vi "From CSV File.vi"(8 "error in (no error)":errorcluster, 9 "Path":path, 10 "engine in":refnum<class "engine configuration.lvclass">, 11 "Modbus Module editor node in":refnum<class "Modbus Module editor node.lvclass">) -> (0 "error out":errorcluster, 1 "Update":bool, 2 "engine out":refnum<class "engine configuration.lvclass">, 3 "Modbus Module editor node out":refnum<class "Modbus Module editor node.lvclass">)   [LabVIEW 2015, in "Modbus Module editor node.lvclass"]
uses:
  Modbus Module editor node.lvclass
  <vilib>/NI/Module Execution Interface/Engine Configuration/engine configuration.lvclass
  module/configuration/Modbus Module configuration.lvclass
  <vilib>/NI/Configuration Framework/serializable configuration/NISE_CEF_serializable configuration.lvclass/NISE_CEF_serializable configuration.ctl
  <vilib>/Utility/LVClass/Get LV Class Name.vi
  <vilib>/NI/Configuration Framework/error generator/NISE_error generator.vi
  <vilib>/NI/Configuration Framework/serializable configuration/NISE_CEF_serializable configuration.lvclass
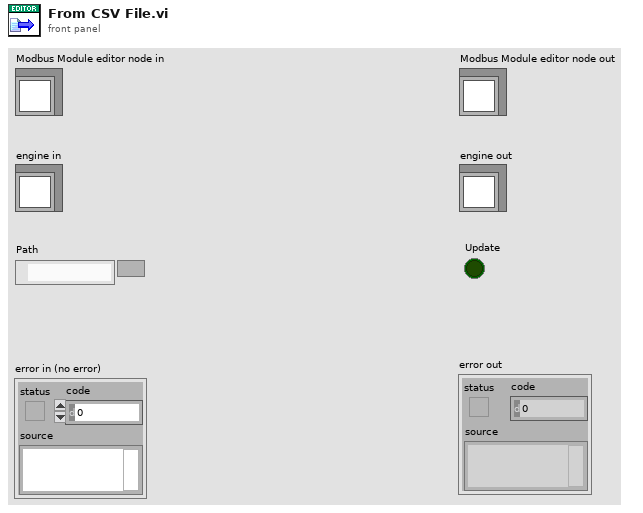
[diagram p1: front panel]
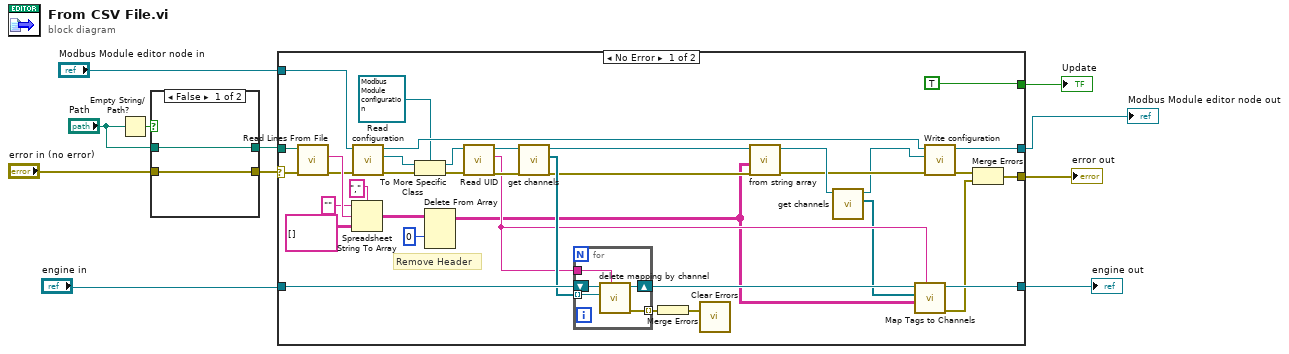
[diagram p0: block diagram]
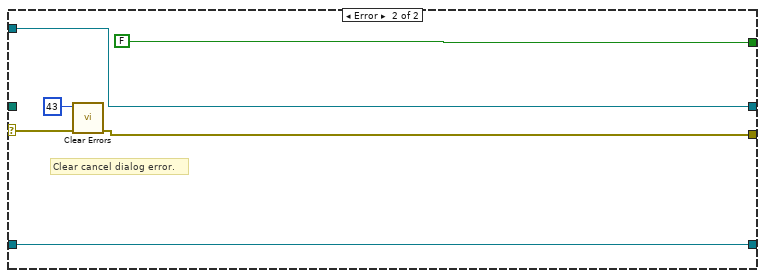
[diagram p2: hidden frame]
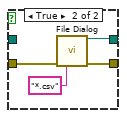
[diagram p3: hidden frame]
diagram:
  n1 = Empty String/Path?(string/path="Path") -> (empty?=w11:bool)
  n2 = case shown="False" w11 {
    tunnel: "error in (no error)" -> [w13 w16]
    tunnel: [w13 w15] -> w9
    tunnel: [w12 w14] -> w10
    tunnel: "Path" -> [w12 _]
    frame False {
    }
    frame True {
      n3 = call "File Dialog"("error in"=w16, "pattern (all files)"="*.csv") -> ("selected path"=w14:path, "error out"=w15:errorcluster)  [unwired: 10 in, 2 out]
    }
  }
  n4 = case shown="No Error" w9 {
    selector: w9 -> [w47 w62]
    tunnel: [w39 w61] -> w2
    tunnel: [w33 w64] -> w5
    tunnel: "Modbus Module editor node in" -> [w38 w64]
    tunnel: w10 -> [w52 _]
    tunnel: [TRUE ("Update") FALSE ("Update")] -> w3
    tunnel: "engine in" -> [w44 w59]
    tunnel: [w25 w59] -> w4
    frame No Error {
      # "Remove Header"
      n5 = call <vilib>:"Read Lines From File.vi"("file path (dialog if empty)"=w52, "error in (not an error)"=w47) -> ("line string"=w50:string, "error out"=w37:errorcluster)  [unwired: 5 in, 1 out]
      n6 = Spreadsheet String To Array(delimiter (Tab)=",", format string="", spreadsheet string=w50, array type (2D Dbl)=string[][] [] ("type (empty)")) -> (array=w20:string[][])
      n7 = call-dynamic "Read configuration.vi"("error in"=w37, "Modbus Slave editor node in"=w38) -> ("error out"=w35:errorcluster, "configuration"=w36:refnum<class "NISE_CEF_serializable configuration.lvclass">, "Modbus Slave editor node out"=w34:refnum<class "Modbus Module editor node.lvclass">)  [unwired: 7 in]
      n8 = To More Specific Class(target class=refnum<class "Modbus Module configuration.lvclass"> refnum ("Modbus Module configuration"), reference=w36, error in=w35) -> (specific class reference=w46:refnum<class "Modbus Module configuration.lvclass">, error out=w40:errorcluster)
      n9 = Delete From Array(array=w20, index (row)=0) -> (array with subset deleted=w19:string[][])  [unwired: 2 in, 1 out]
      n10 = call <vilib>:"Read UID.vi"("error in"=w40, "configuration in"=w46) -> ("error out"=w30:errorcluster, "instance id"=w22:string, "configuration out"=w45:refnum<class "Modbus Module configuration.lvclass">)  [unwired: 7 in]
      n11 = call-dynamic "get channels.vi"("Modbus Slave configuration in"=w45) -> ("channels"=w43:refnum<class "TBM channel.lvclass">[], "Modbus Slave configuration out"=w41:refnum<class "Modbus Module configuration.lvclass">)  [unwired: 9 in]
      n12 = for {
        tunnel: w22 -> [w57]
        tunnel: w43 -> [w56] mode=indexing
        tunnel: [w55] -> w42 mode=indexing
        shift-right: [w54] -> w24
        shift-left: w44 -> [w58]
        n13 = call <vilib>:"delete mapping by channel.vi"("owner ID"=w57, "channel"=w56, "engine configuration in"=w58) -> ("error out"=w55:errorcluster, "engine configuration out"=w54:refnum<class "engine configuration.lvclass">)  [unwired: 7 in]
      }
      n14 = Merge Errors(w42) -> (w31:errorcluster)
      n15 = call <vilib>:"Clear Errors.vi"("error in (no error)"=w31) -> ()  [unwired: 5 in, 2 out]
      n16 = call-dynamic "from string array.vi"("error in (no error)"=w30, "String Array"=w19, "module configuration in"=w41) -> ("error out"=w27:errorcluster, "module configuration out"=w28:refnum<class "Modbus Module configuration.lvclass">)  [unwired: 7 in]
      n17 = call-dynamic "get channels.vi"("Modbus Slave configuration in"=w28) -> ("channels"=w21:refnum<class "TBM channel.lvclass">[], "Modbus Slave configuration out"=w26:refnum<class "Modbus Module configuration.lvclass">)  [unwired: 9 in]
      n18 = call "Map Tags to Channels.vi"("instance id"=w22, "String Array"=w19, "channels"=w21, "engine configuration in"=w24) -> ("error out"=w23:errorcluster, "engine configuration out"=w25:refnum<class "engine configuration.lvclass">)  [unwired: 6 in]
      n19 = call-dynamic "Write configuration.vi"("error in"=w27, "configuration"=w26, "Modbus Slave editor node in"=w34) -> ("error out"=w32:errorcluster, "Modbus Slave editor node out"=w33:refnum<class "Modbus Module editor node.lvclass">)  [unwired: 7 in]
      n20 = Merge Errors(w32, w23) -> (w39:errorcluster)
    }
    frame Error {
      # "Clear cancel dialog error."
      n21 = call <vilib>:"Clear Errors.vi"("error in (no error)"=w62, "specific error code to clear (0: all)"=43) -> ("error out"=w61:errorcluster)  [unwired: 4 in, 1 out]
    }
  }
  "error out" <- w2
  "Modbus Module editor node out" <- w5
  "Update" <- w3
  "engine out" <- w4
